vi "Error Time Check.vi"(9 "Ticks Until Trigger":u32=400000000, 11 "Limit Exceeded":bool) -> (3 "Limit Triggered":bool)   [LabVIEW 2018]
doc: "Author: Scott Hannahs <sth@magnet.fsu.edu>\nCopyright 2018 Florida State University, All rights reserved."
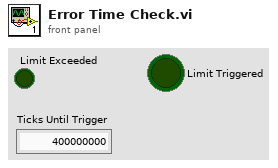
[diagram p1: front panel]
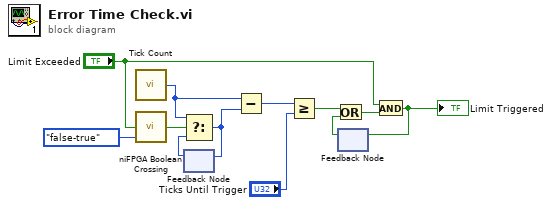
[diagram p0: block diagram]
diagram:
  n1 = call "Tick Count"() -> ("Tick Count(Ticks)"=w7:u32)
  n2 = call <vilib>:"niFPGA Boolean Crossing.vi"("input"="Limit Exceeded", "direction"=enum8{"either", "false-true", "true-false"}."false-true") -> ("crossing"=w9:bool)  [unwired: 7 in]
  n3 = feedback #1() -> (w8:u32)  [unwired: 1 in]
  n4 = Select(t=w7, s=w9, f=w8) -> (s? t:f=w6:u32)
  n5 = feedback-in #1(w6) -> ()
  n6 = Subtract(x=w7, y=w6) -> (x-y=w5:u32)
  n7 = Greater Or Equal?(x=w5, y="Ticks Until Trigger") -> (x >= y?=w4:bool)
  n8 = feedback #2() -> (w3:bool)  [unwired: 1 in]
  n9 = Or(x=w4, y=w3) -> (x .or. y?=w2:bool)
  n10 = And(x="Limit Exceeded", y=w2) -> (x .and. y?=w1:bool)
  "Limit Triggered" <- w1
  n11 = feedback-in #2(w1) -> ()
